vi "On Compile - Group Hardware Channels by Message Type.vi"(8 "error in":errorcluster, 11 "hardware channel data":T2[](array[typedef]) {"labels settings for RT"."Label Timestamp Channel Data Reference" format="%.0x"; "labels settings for RT"."Word Initial Raw Value" format="%032.0f"; "labels settings for RT"."Label Disable/Trigger Channel Reference" format="%.0x"; "labels settings for RT"."parameter driver data"."Tx parameter refs" format="%.0x"; "labels settings for RT"."parameter driver data"."Rx block data refs"."Data Reference" format="%.0x"; "labels settings for RT"."SDI" format="%02b"; "labels settings for RT"."label" format="%.0o"}) -> (0 "error out":errorcluster, 3 "grouped hardware channel data refs":T11(array[cluster]) {"hardware channel data"."labels settings for RT"."Label Timestamp Channel Data Reference" format="%.0x"; "hardware channel data"."labels settings for RT"."Word Initial Raw Value" format="%032.0f"; "hardware channel data"."labels settings for RT"."Label Disable/Trigger Channel Reference" format="%.0x"; "hardware channel data"."labels settings for RT"."parameter driver data"."Tx parameter refs" format="%.0x"; "hardware channel data"."labels settings for RT"."SDI" format="%02b"; "hardware channel data"."labels settings for RT"."label" format="%.0o"; "VS Refs" format="%.0x"})   [LabVIEW 2020, in "Ballard ARINC 429 System Explorer.lvlib" / "Implementation.lvlib"]
uses:
  Implementation.lvlib
  Shared/RT Hardware Channel Settings.ctl
  Shared/RT Label Settings.ctl
  Shared/Label.ctl
  Shared/RT Parameters.ctl
  Shared/Parameter Definition.ctl
  Encoding and Decoding/Encoding.ctl
  <vilib>/NI VeriStand/Custom Device API/Block Data Reference.ctl
  <vilib>/NI VeriStand/Custom Device API/Data Reference.ctl
  <vilib>/NI VeriStand/Custom Device API/Custom Device Item Ref.ctl
  Shared/Transfer Type.ctl
  <vilib>/NI VeriStand/Custom Device API/Custom Device API.lvlib
  Encoding and Decoding/Encoding and Decoding.lvlib
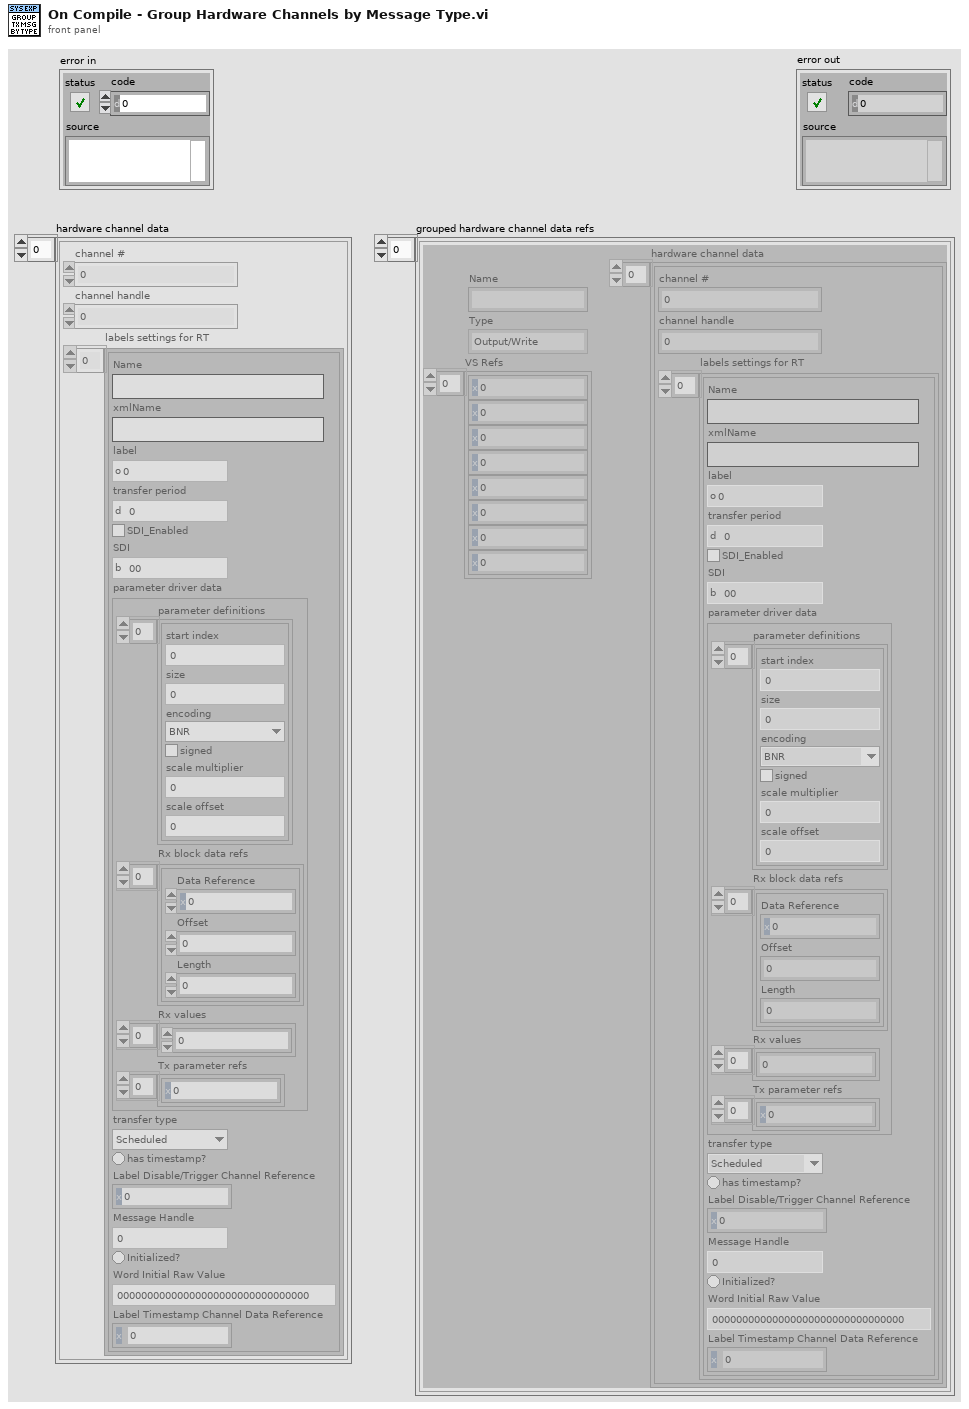
[diagram p1: front panel]
types:
  T1 = typedef "Custom Device API.lvlib/Custom Device Item Ref.ctl" = u64
  T2 = typedef "RT Hardware Channel Settings.ctl" = cluster{"channel #":u16, "channel handle":u64, "labels settings for RT":T3[]}
  T3 = typedef "RT Label Settings.ctl" = cluster{"Name":string, "xmlName":string, "label":T4, "transfer period":u32, "SDI_Enabled":bool, "SDI":u8, "parameter driver data":T5, "transfer type":T10, "has timestamp?":bool, "Label Disable/Trigger Channel Reference":T1, "Message Handle":u64, "Initialized?":bool, "Word Initial Raw Value":u32, "Label Timestamp Channel Data Reference":T9}
  T4 = typedef "Label.ctl" = u8
  T5 = typedef "RT Parameters.ctl" = cluster{"parameter definitions":T6[], "Rx block data refs":T8[], "Rx values":dbl[], "Tx parameter refs":T1[]}
  T6 = typedef "Parameter Definition.ctl" = cluster{"start index":i32, "size":i32, "encoding":T7, "signed":bool, "scale multiplier":dbl, "scale offset":dbl}
  T7 = typedef "Encoding and Decoding.lvlib/Encoding.ctl" = enum16{"BNR", "BCD", "Discrete"}
  T8 = typedef "Custom Device API.lvlib/Block Data Reference.ctl" = cluster{"Data Reference":T9, "Offset":u64, "Length":u64}
  T9 = typedef "Custom Device API.lvlib/Data Reference.ctl" = i32
  T10 = typedef "Transfer Type.ctl" = enum16{"Scheduled", "Acyclic", "Block", "Strobe"}
  T11 = cluster{"Name":string, "Type":enum16{"Output/Write", "Input/Read", "Input/ReadWrite"}, "VS Refs":T1[], "hardware channel data":T2[]}[]
  T12 = cluster{"Group":cluster{"Name":string, "Type":enum16{"Output/Write", "Input/Read", "Input/ReadWrite"}, "VS Refs":T1[], "hardware channel data":T2[]}, "transfer type":T10}[]
  T13 = cluster{"Name":string, "Type":enum16{"Output/Write", "Input/Read", "Input/ReadWrite"}, "VS Refs":T1[], "hardware channel data":T2[]}
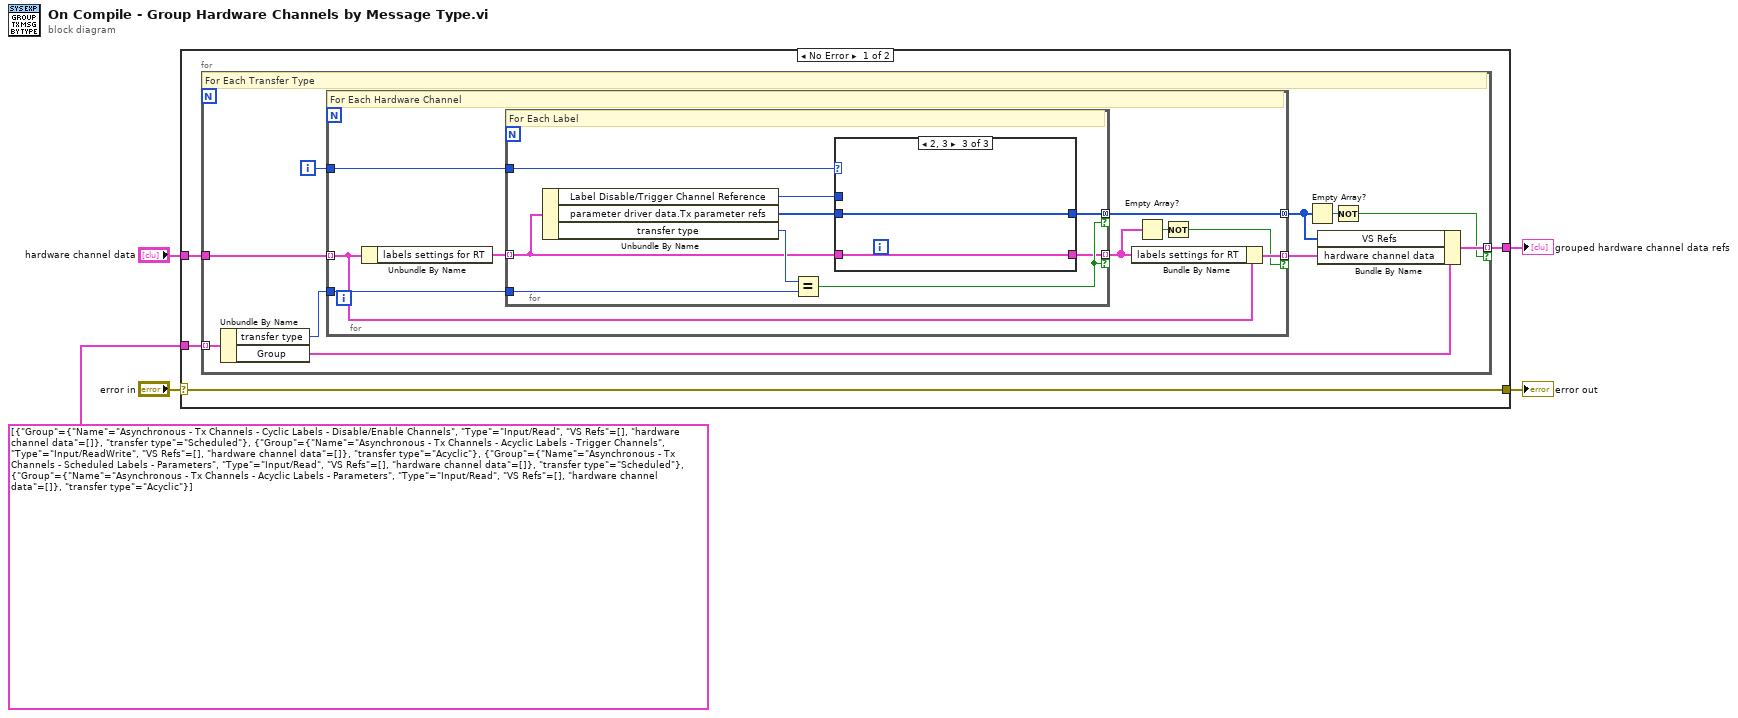
[diagram p0: block diagram]
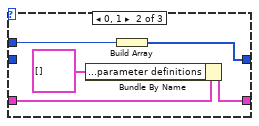
[diagram p3: hidden frame]
diagram:
  n1 = case shown="No Error" "error in" {
    selector: "error in" -> [w8 w46]
    tunnel: "hardware channel data" -> [w9 _]
    tunnel: [w8 w46] -> w3
    tunnel: T12 [{"Group"={"Name"="Asynchronous - Tx Channels - Cyclic Labels - Disable/Enable Channels", "Type"=enum."Input/Read", "VS Refs"=[], "hardware channel data"=[]}, "transfer type"=enum."Scheduled"}, {"Group"={"Name"="Asynchronous - Tx Channels - Acyclic Labels - Trigger Channels", "Type"=enum."Input/ReadWrite", "VS Refs"=[], "hardware channel data"=[]}, "transfer type"=enum."Acyclic"}, {"Group"={"Name"="Asynchronous - Tx Channels - Scheduled Labels - Parameters", "Type"=enum."Input/Read", "VS Refs"=[], "hardware channel data"=[]}, "transfer type"=enum."Scheduled"}, {"Group"={"Name"="Asynchronous - Tx Channels - Acyclic Labels - Parameters", "Type"=enum."Input/Read", "VS Refs"=[], "hardware channel data"=[]}, "transfer type"=enum."Acyclic"}] -> [w7 _]
    tunnel: [w6 _] -> w2
    frame No Error {
      n2 = for {
        tunnel: w9 -> [w19]
        tunnel: w7 -> [w18] mode=indexing
        tunnel: [w15] -> w6 mode=indexing if=w12
        i -> [w16]
        # "For Each Transfer Type"
        n3 = Unbundle By Name(w18) -> ("transfer type"=w17:T10, "Group"=w10:T13)
        n4 = for {
          tunnel: w19 -> [w24] mode=indexing
          tunnel: w17 -> [w27]
          tunnel: w16 -> [w26]
          tunnel: [w25] -> w14 mode=concatenating
          tunnel: [w23] -> w11 mode=indexing if=w20
          # "For Each Hardware Channel"
          n5 = Unbundle By Name(w24) -> ("labels settings for RT"=w28:T3[])
          n6 = for {
            tunnel: w28 -> [w29] mode=indexing
            tunnel: w27 -> [w36]
            tunnel: w26 -> [w35]
            tunnel: [w34] -> w25 mode=concatenating if=w31
            tunnel: [w30] -> w21 mode=indexing if=w31
            # "For Each Label"
            n7 = Unbundle By Name(w29) -> ("Label Disable/Trigger Channel Reference"=w33:T1, "parameter driver data.Tx parameter refs"=w32:T1[], "transfer type"=w37:T10)
            n8 = Equal?(x=w37, y=w36) -> (x = y?=w31:bool)
            n9 = case shown="2, 3" w35 {
              tunnel: [_ w43 w45] -> w34
              tunnel: w33 -> [_ w42 _]
              tunnel: w32 -> [_ _ w45]
              tunnel: [w38 w40 w44] -> w30
              tunnel: w29 -> [w38 w41 w44]
              frame Default {
              }
              frame 0, 1 {
                n10 = Bundle By Name(cluster=w41, "parameter driver data.parameter definitions"=T6[] []) -> (w40:T3)
                n11 = Build Array(w42) -> (w43:T1[])
              }
              frame 2, 3 {
              }
            }
          }
          n12 = Bundle By Name(cluster=w24, "labels settings for RT"=w21) -> (w23:T2)
          n13 = Empty Array?(array=w21) -> (empty?=w22:bool)
          n14 = Not(x=w22) -> (.not. x?=w20:bool)
        }
        n15 = Empty Array?(array=w14) -> (empty?=w13:bool)
        n16 = Bundle By Name(cluster=w10, "VS Refs"=w14, "hardware channel data"=w11) -> (w15:T13)
        n17 = Not(x=w13) -> (.not. x?=w12:bool)
      }
    }
    frame Error {
    }
  }
  "error out" <- w3
  "grouped hardware channel data refs" <- w2
